vi "TestOPC.vi"() -> ()   [LabVIEW 2020]
panel:
  out "error out":errorcluster
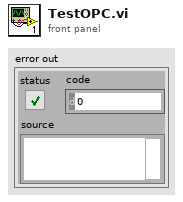
[diagram p1: front panel]
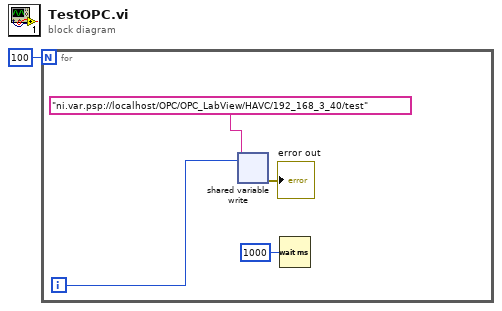
[diagram p0: block diagram]
diagram:
  n1 = for {
    N: 100 -> [_]
    i -> [w3]
    n2 = shared-variable-write("ni.var.psp://localhost/OPC/OPC_LabView/HAVC/192_168_3_40/test", w3) -> (→"error out":errorcluster)  [unwired: 1 in, 1 out]
    n3 = Wait (ms)(milliseconds to wait=u32 1000) -> ()  [unwired: 1 out]
  }
